vi "Set Fast Kinetics Ex.vi"(4 "offset":i32, 5 "vbin":i32, 6 "hbin":i32, 7 "mode":i32, 9 "time":sgl, 10 "seriesLength":i32, 11 "exposedRows":i32) -> (3 "function return":u32)   [LabVIEW 2018, in "Copy of Andor SDK.lvlib"]
doc: "EXPNETTYPE unsigned int WINAPI SetFastKineticsEx(int exposedRows, int seriesLength, float time, int mode, int hbin, int vbin, int offset);"
uses:
  Copy of Andor SDK.lvlib
  <userlib>/Andor SDK/ATMCD32D.dll
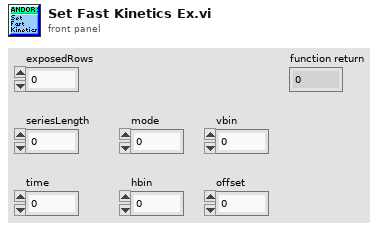
[diagram p1: front panel]
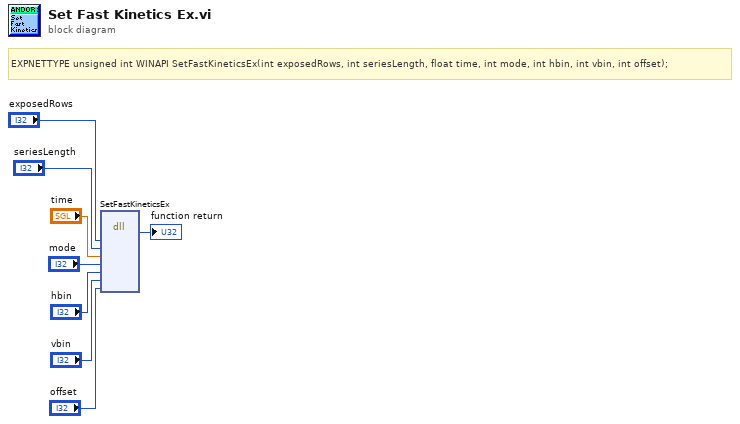
[diagram p0: block diagram]
diagram:
  # "EXPNETTYPE unsigned int WINAPI SetFastKineticsEx(int exposedRows, int seriesLength, float time, int mode, int hbin, int vbin, int offset);"
  n1 = dll-call lib="C:/Program Files (x86)/National Instruments/LabVIEW 2018/user.lib/Andor SDK/ATMCD32D.*" fn="SetFastKineticsEx"("exposedRows"="exposedRows", "seriesLength"="seriesLength", "time"="time", "mode"="mode", "hbin"="hbin", "vbin"="vbin", "offset"="offset") -> (→"function return":u32)  [unwired: 10 in, 2 out]
